vi "Coordenadas_Int_a_Coordenadas_Str.vi"(1 "Columna":dbl, 2 "Fila":dbl) -> (0 "Posicion_str":string)   [LabVIEW 2019]
doc: "Convierte las posición de fila y columna en una coordena 'x,y' de tipo String."
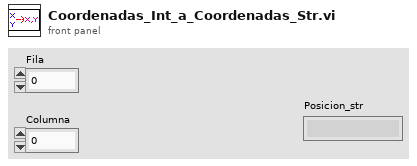
[diagram p1: front panel]
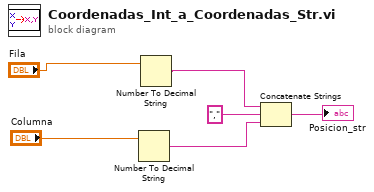
[diagram p0: block diagram]
diagram:
  n1 = Number To Decimal String(number="Columna") -> (decimal integer string=w2:string)  [unwired: 1 in]
  n2 = Number To Decimal String(number="Fila") -> (decimal integer string=w3:string)  [unwired: 1 in]
  n3 = Concatenate Strings(w3, "," ("string"), w2) -> (→"Posicion_str":string)
